vi "setVertSettingsDevice.vi"(8 "error in (no error)":errorcluster, 9 "Channels":string, 10 "Channel settings":T1, 11 "IVI Refnum in":refnum<k15>) -> (0 "error out":errorcluster, 2 "Channel settings out":T1, 3 "IVI Refnum out":refnum<k15>)   [LabVIEW 2011]
uses:
  ChannelSettings_TypDef.ctl
  coupling_Enum_TypDef.ctl
  impedance_Enum_TypDEf.ctl
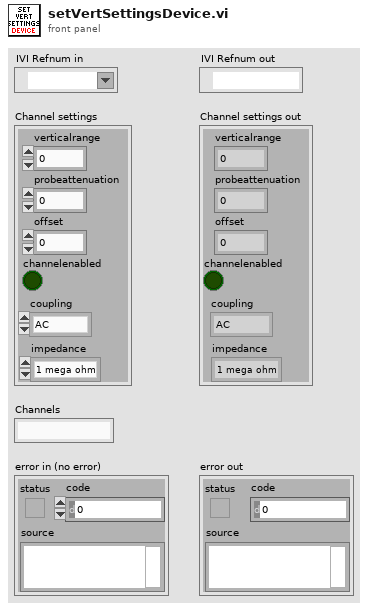
[diagram p1: front panel]
types:
  T1 = typedef "ChannelSettings_TypDef.ctl" = cluster{"verticalrange":dbl, "probeattenuation":dbl, "offset":dbl, "channelenabled":bool, "coupling":T2, "impedance":T3}
  T2 = typedef "coupling_Enum_TypDef.ctl" = enum16{"AC", "DC", "Ground"}
  T3 = typedef "impedance_Enum_TypDEf.ctl" = enum16{"1 mega ohm", "<NA>", "50 ohms"}
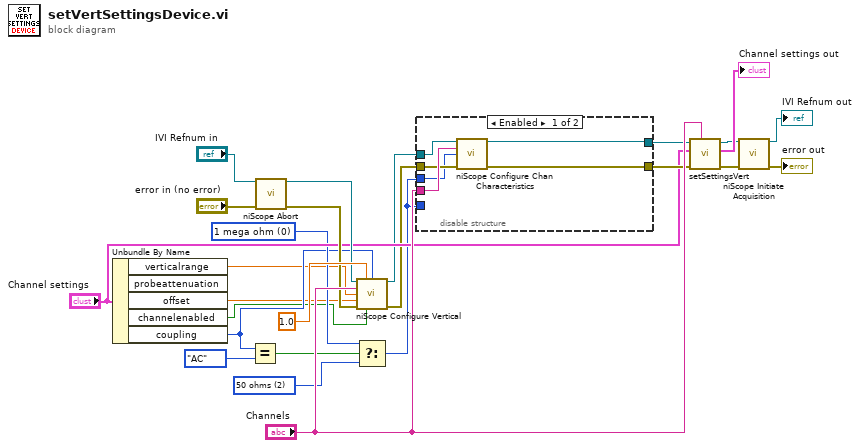
[diagram p0: block diagram]
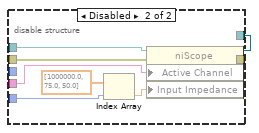
[diagram p2: hidden frame]
diagram:
  w10 = u32 2 items=["1 mega ohm"=0, "50 ohms"=2] ("input impedance")
  w9 = u32 0 items=["1 mega ohm"=0, "50 ohms"=2] ("input impedance")
  n1 = Unbundle By Name("Channel settings") -> ("verticalrange"=w3:dbl, "offset"=w4:dbl, "channelenabled"=w5:bool, "coupling"=w6:T2)  [unwired: 1 out]
  n2 = Equal?(x=w6, y=coupling_Enum_TypDef."AC") -> (x = y?=w8:bool)
  n3 = call "niScope Abort.vi"("instrument handle"="IVI Refnum in", "error in"="error in (no error)") -> ("instrument handle out"=w23:refnum<k15>, "error out"=w21:errorcluster)  [unwired: 12 in]
  n4 = call "niScope Configure Vertical.vi"("instrument handle"=w23, "probe attenuation"=1.0, "vertical coupling"=w6, "channels"="Channels", "vertical range"=w3, "vertical offset"=w4, "error in"=w21, "channel enabled"=w5) -> ("instrument handle out"=w2:refnum<k15>, "error out"=w11:errorcluster)  [unwired: 6 in]
  n5 = Select(t=w9, s=w8, f=w10) -> (s? t:f=w1:u32)
  n6 = disable-structure shown="Enabled" {
    disable-tunnel: "Channels" -> [w31 w37]
    disable-tunnel: [w30 w32] -> w22
    disable-tunnel: [w29 w38] -> w16
    disable-tunnel: w11 -> [w28 w33]
    disable-tunnel: w1 -> [w27 _]
    disable-tunnel: w2 -> [w26 w39]
    disable-tunnel: w1 -> [_ w35]
    frame Enabled {
      n7 = call "niScope Configure Chan Characteristics.vi"("instrument handle"=w26, "channels"=w31, "input impedance"=w27, "error in"=w28) -> ("instrument handle out"=w29:refnum<k15>, "error out"=w30:errorcluster)  [unwired: 1 in, 9 out]
    }
    frame Disabled {
      n8 = Index Array(array=dbl[] [1000000.0, 75.0, 50.0] ("input impedance arr"), index=w35) -> (element=w34:dbl)
      n9 = property class="niScope"(reference=w39, error in=w33, "Active Channel"=w37, "Input Impedance"=w34) -> (reference out=w38:refnum<k15>, error out=w32:errorcluster)
    }
  }
  n10 = call "setSettingsVert.vi"("Active Channel"="Channels", "error out in"=w22, "Channel settings"="Channel settings", "IVI Refnum in"=w16) -> ("error out out"=w18:errorcluster, "Channel settings out"=→"Channel settings out":T1, "IVI Refnum out"=w13:refnum<k15>)  [unwired: 5 in]
  n11 = call "niScope Initiate Acquisition.vi"("instrument handle"=w13, "error in"=w18) -> ("instrument handle out"=→"IVI Refnum out":refnum<k15>, "error out"=→"error out":errorcluster)  [unwired: 12 in]
